vi "Get Pulsar Info.vi"(8 "error in":errorcluster, 11 "OphirFastX (in)":refnum<k7>) -> (0 "error out":errorcluster, 2 "Pulsar Handle":i16, 3 "OphirFastX (out)":refnum<k7>, 4 "Device Found?":bool, 5 "Pulsar Info":string)   [LabVIEW 2009]
panel:
  # "Guillaume Plateau - yguig2@yahoo.fr"
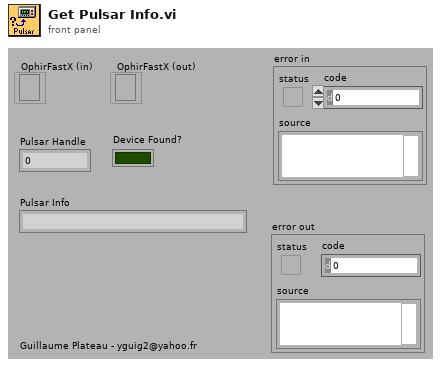
[diagram p1: front panel]
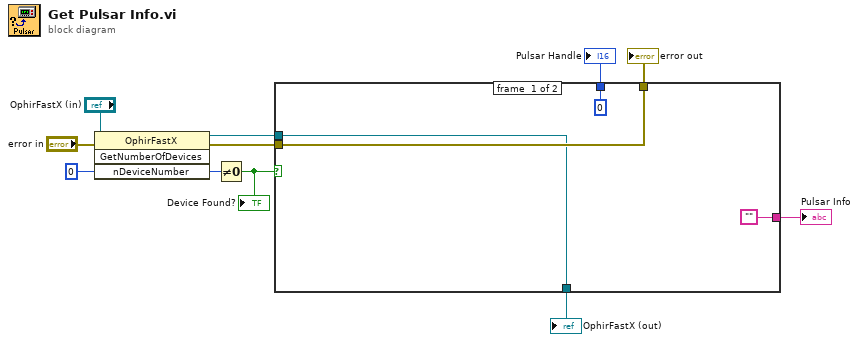
[diagram p0: block diagram]
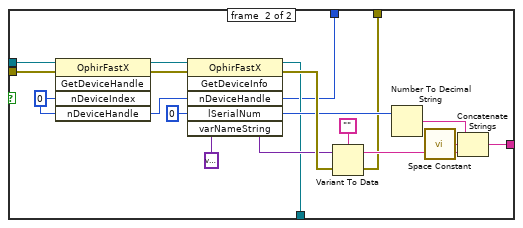
[diagram p2: hidden frame]
diagram:
  n1 = invoke class="OphirFastX" method="GetNumberOfDevices"(reference="OphirFastX (in)", error in="error in", "nDeviceNumber"=i16 0) -> (reference out=w7:refnum<k7>, error out=w8:errorcluster, "nDeviceNumber"=w6:i16)  [unwired: 1 in, 1 out]
  n2 = Not Equal To 0?(x=w6) -> (x != 0?=w10:bool)
  "Device Found?" <- w10
  n3 = case shown="True" w10 {
    tunnel: w7 -> [w14 w34]
    tunnel: w8 -> [w15 w33]
    tunnel: [w15 w19] -> w2
    tunnel: [w14 w18] -> w1
    tunnel: ["" w17] -> w9
    tunnel: [i16 0 ("nDeviceHandle") w16] -> w11
    frame #0 {
    }
    frame #1 {
      w32 = i16 0 ("nDeviceIndex")
      n4 = invoke class="OphirFastX" method="GetDeviceHandle"(reference=w34, error in=w33, "nDeviceIndex"=w32, "nDeviceHandle"=w32) -> (reference out=w31:refnum<k7>, error out=w30:errorcluster, "nDeviceHandle"=w29:i16)  [unwired: 1 in, 2 out]
      n5 = invoke class="OphirFastX" method="GetDeviceInfo"(reference=w31, error in=w30, "nDeviceHandle"=w29, "lSerialNum"=0, "varNameString"=variant) -> (reference out=w18:refnum<k7>, error out=w26:errorcluster, "nDeviceHandle"=w16:i16, "lSerialNum"=w23:i32, "varNameString"=w24:variant)  [unwired: 1 in, 1 out]
      n6 = Variant To Data(error in=w26, Variant=w24, type="") -> (error out=w19:errorcluster, data=w22:string)
      n7 = Number To Decimal String(number=w23) -> (decimal integer string=w21:string)  [unwired: 1 in]
      n8 = call <vilib>:"Space Constant.vi"() -> ("String"=w20:string)
      n9 = Concatenate Strings(w21, w20, w22) -> (w17:string)
    }
  }
  "Pulsar Handle" <- w11
  "Pulsar Info" <- w9
  "OphirFastX (out)" <- w1
  "error out" <- w2
